vi "Tokens to Object.vi"(8 "error in":errorcluster, 10 "starting index":i32, 11 "array w/ subset deleted":cluster{"Token Type":T1, "Token Value":string}[](array[cluster])) -> (0 "error out":errorcluster, 2 "next index":i32, 3 "JSON Object out":refnum<class "JSON Object.lvclass">)   [LabVIEW 2015, in "LVJSON.lvlib" / "JSON Helper.lvclass"]
uses:
  JSON Data Classes/JSON Helper/JSON Helper.lvclass
  JSON Data Classes/JSON Object/JSON Object.lvclass
  Token Types.ctl
  JSON Data Classes/JSON Object/New JSON Object (Multi).vi
  JSON Data Classes/JSON String/New JSON String.vi
  JSON Data Classes/JSON Datatype/New JSON Null.vi
  JSON Data Classes/JSON Boolean/New JSON Boolean.vi
  JSON Data Classes/JSON Numeric/New JSON Numeric.vi
  JSON Data Classes/JSON String/JSON String.lvclass
  JSON Data Classes/JSON Datatype/JSON Null.lvclass
  JSON Data Classes/JSON Boolean/JSON Boolean.lvclass
  JSON Data Classes/JSON Numeric/JSON Numeric.lvclass
  LVJSON.lvlib
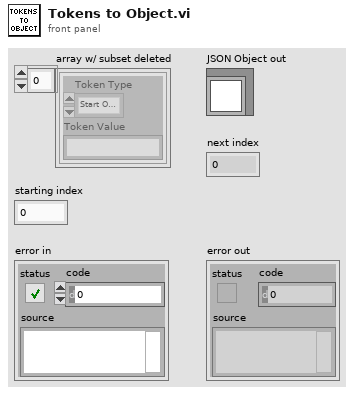
[diagram p1: front panel]
types:
  T1 = typedef "LVJSON.lvlib/Token Types.ctl" = enum32{"Start Object", "End Object", "Start Array", "End Array", "Quotation", "Numeric", "true", "false", "null", "Escape", "Undefined"}
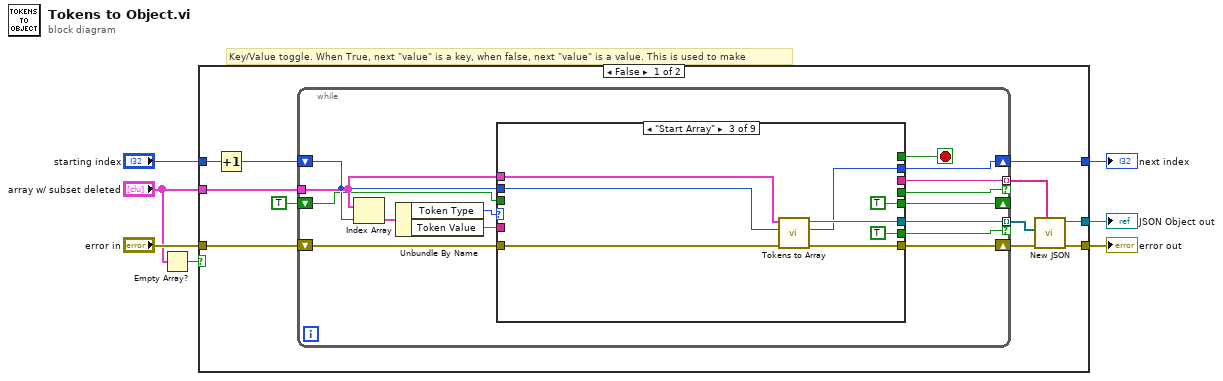
[diagram p0: block diagram]
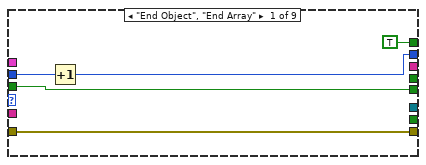
[diagram p2: hidden frame]
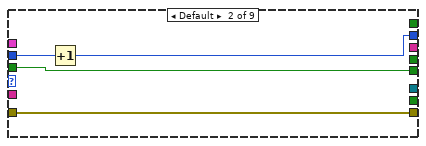
[diagram p3: hidden frame]
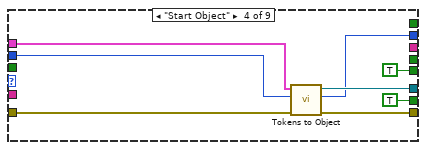
[diagram p4: hidden frame]
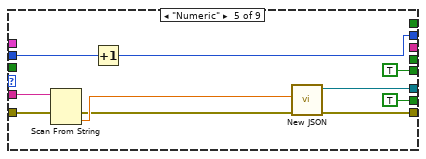
[diagram p5: hidden frame]
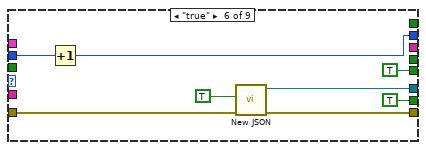
[diagram p6: hidden frame]
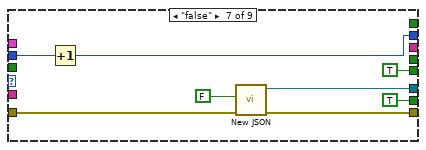
[diagram p7: hidden frame]
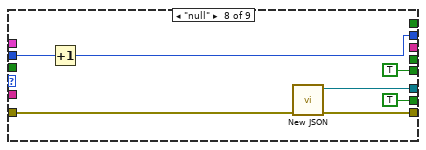
[diagram p8: hidden frame]
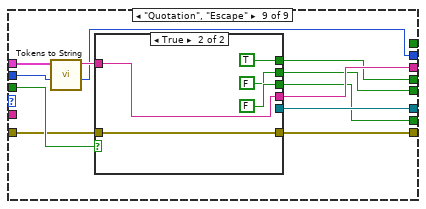
[diagram p9: hidden frame]
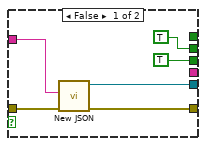
[diagram p10: hidden frame]
diagram:
  # "Key/Value toggle. When True, next \"value\" is a key, when false, next \"value\" is a value. This is used to make"
  n1 = Empty Array?(array="array w/ subset deleted") -> (empty?=w1:bool)
  n2 = case shown="False" w1 {
    tunnel: [w12 _] -> w7
    tunnel: "array w/ subset deleted" -> [w18 _]
    tunnel: "error in" -> [w17 w115]
    tunnel: [w10 w115] -> w5
    tunnel: [w14 w116] -> w4
    tunnel: "starting index" -> [w13 w116]
    frame False {
      n3 = Increment(x=w13) -> (x+1=w15:i32)
      n4 = while {
        tunnel: w18 -> [w26]
        tunnel: [w30] -> w8 mode=indexing if=w19
        shift-right: [w25] -> w14
        shift-left: w15 -> [w24]
        shift-right: [w27] -> w16
        shift-left: w17 -> [w28]
        shift-right: [w20] -> _
        shift-left: TRUE -> [w23]
        tunnel: [w22] -> w9 mode=indexing if=w21
        stop <- w31 stop-if-true
        n5 = Index Array(array=w26, index=w24) -> (element=w29:cluster{"Token Type":T1, "Token Value":string})
        n6 = Unbundle By Name(w29) -> ("Token Type"=w33:T1, "Token Value"=w32:string)
        n7 = case shown="\"Start Array\"" w33 {
          tunnel: w32 -> [_ _ _ _ w67 _ _ _ _]
          tunnel: [TRUE _ _ _ _ _ _ _ _] -> w31
          tunnel: [_ _ w47 w55 w68 w75 w83 w91 w103] -> w30
          tunnel: [_ _ TRUE TRUE TRUE TRUE TRUE TRUE w97] -> w19
          tunnel: w28 -> [w38 w42 w50 w58 w64 w73 w81 w89 w96]
          tunnel: [w38 w42 w49 w57 w62 w72 w80 w88 w102] -> w27
          tunnel: w26 -> [_ _ w48 w56 _ _ _ _ w95]
          tunnel: w24 -> [w37 w41 w44 w52 w61 w71 w79 w87 w94]
          tunnel: [w36 w40 w45 w53 w60 w70 w78 w86 w92] -> w25
          tunnel: w23 -> [w34 w39 _ _ _ _ _ _ w101]
          tunnel: [w34 w39 TRUE TRUE TRUE TRUE TRUE TRUE w98] -> w20
          tunnel: [_ _ _ _ _ _ _ _ w100] -> w22
          tunnel: [_ _ _ _ _ _ _ _ w99] -> w21
          frame "End Object", "End Array" {
            n8 = Increment(x=w37) -> (x+1=w36:i32)
          }
          frame Default {
            n9 = Increment(x=w41) -> (x+1=w40:i32)
          }
          frame "Start Array" {
            n10 = call "Tokens to Array.vi"("error in"=w50, "starting index"=w44, "array w/ subset deleted"=w48) -> ("error out"=w49:errorcluster, "next index"=w45:i32, "JSON Array out"=w47:refnum<class "JSON Array.lvclass">)  [unwired: 6 in]
          }
          frame "Start Object" {
            n11 = call "Tokens to Object.vi"("error in"=w58, "starting index"=w52, "array w/ subset deleted"=w56) -> ("error out"=w57:errorcluster, "next index"=w53:i32, "JSON Object out"=w55:refnum<class "JSON Object.lvclass">)  [unwired: 6 in]
          }
          frame "Numeric" {
            n12 = Scan From String(input string=w67, error in=w64) -> (error out=w63:errorcluster, output 1=w66:dbl)  [unwired: 3 in, 2 out]
            n13 = Increment(x=w61) -> (x+1=w60:i32)
            n14 = call-poly "New JSON.vi"("error in (no error)"=w63, "value"=w66) -> ("error out"=w62:errorcluster, "JSON String out"=w68:refnum<class "JSON Numeric.lvclass">)  [unwired: 8 in]
          }
          frame "true" {
            n15 = Increment(x=w71) -> (x+1=w70:i32)
            n16 = call-poly "New JSON.vi"("error in (no error)"=w73, "value"=TRUE) -> ("error out"=w72:errorcluster, "JSON String out"=w75:refnum<class "JSON Boolean.lvclass">)  [unwired: 8 in]
          }
          frame "false" {
            n17 = Increment(x=w79) -> (x+1=w78:i32)
            n18 = call-poly "New JSON.vi"("error in (no error)"=w81, "value"=FALSE) -> ("error out"=w80:errorcluster, "JSON String out"=w83:refnum<class "JSON Boolean.lvclass">)  [unwired: 8 in]
          }
          frame "null" {
            n19 = Increment(x=w87) -> (x+1=w86:i32)
            n20 = call-poly "New JSON.vi"("error in (no error)"=w89) -> ("error out"=w88:errorcluster, "JSON Null out"=w91:refnum<class "JSON Null.lvclass">)  [unwired: 9 in]
          }
          frame "Quotation", "Escape" {
            n21 = call "Tokens to String.vi"("start index"=w94, "Value Tokens"=w95) -> ("next index"=w92:i32, "String Value"=w93:string)  [unwired: 7 in, 1 out]
            n22 = case shown="True" w101 {
              tunnel: [w109 _] -> w103
              tunnel: w93 -> [w108 w112]
              tunnel: w96 -> [w107 w113]
              tunnel: [w106 w113] -> w102
              tunnel: [TRUE FALSE] -> w97
              tunnel: [_ w112] -> w100
              tunnel: [_ TRUE] -> w99
              tunnel: [TRUE FALSE] -> w98
              frame False {
                n23 = call-poly "New JSON.vi"("error in (no error)"=w107, "value"=w108) -> ("error out"=w106:errorcluster, "JSON String out"=w109:refnum<class "JSON String.lvclass">)  [unwired: 8 in]
              }
              frame True {
              }
            }
          }
        }
      }
      n24 = call-poly "New JSON.vi"("keys"=w9, "error in (no error)"=w16, "values"=w8) -> ("error out"=w10:errorcluster, "JSON Object out"=w12:refnum<class "JSON Object.lvclass">)  [unwired: 7 in]
    }
    frame True {
    }
  }
  "next index" <- w4
  "JSON Object out" <- w7
  "error out" <- w5
